vi "Read ID.vi"(8 "error in (no error)":errorcluster, 11 "8846A in":refnum<class "8846A.lvclass">) -> (0 "error out":errorcluster, 3 "8846A out":refnum<class "8846A.lvclass">)   [LabVIEW 2015, in "8846A.lvclass"]
doc: "VI used to Read Hardware ID"
uses:
  8846A.lvclass
  <instrlib>/Fluke 884X Series/Fluke 884X Series.lvlib
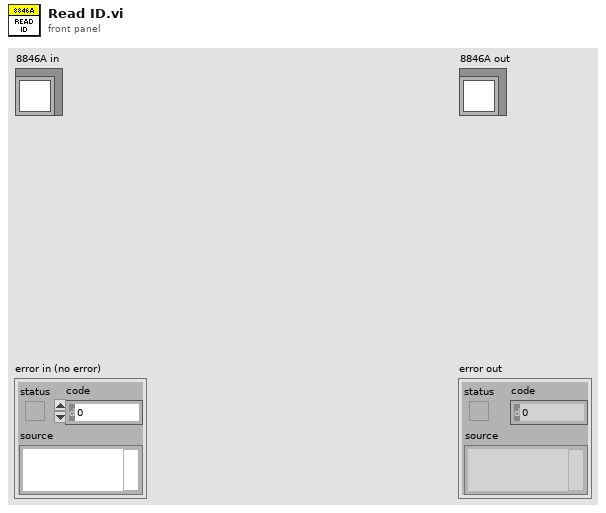
[diagram p1: front panel]
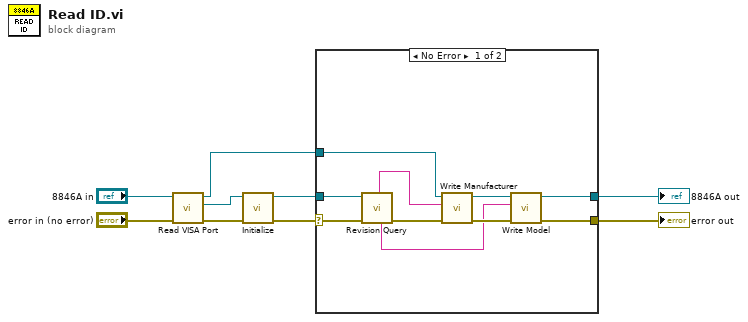
[diagram p0: block diagram]
diagram:
  n1 = call-dynamic "Read VISA Port.vi"("error in (no error)"="error in (no error)", "Device in"="8846A in") -> ("error out"=w8:errorcluster, "VISA Port"=w9:refnum<visa-resource-name>, "Device out"=w5:refnum<class "8846A.lvclass">)  [unwired: 7 in]
  n2 = call <instrlib>:"Initialize.vi"("error in (no error)"=w8, "VISA resource name"=w9) -> ("error out"=w6:errorcluster, "VISA resource name out"=w7:refnum<visa-resource-name>)  [unwired: 8 in]
  n3 = case shown="No Error" w6 {
    selector: w6 -> [w10 w20]
    tunnel: w7 -> [w19 _]
    tunnel: w5 -> [w18 w21]
    tunnel: [w12 w20] -> w1
    tunnel: [w11 w21] -> w2
    frame No Error {
      n4 = call <instrlib>:"Revision Query.vi"("error in (no error)"=w10, "VISA resource name"=w19) -> ("error out"=w16:errorcluster, "Modelo"=w13:string, "Fabricante"=w17:string)  [unwired: 4 in, 3 out]
      n5 = call-dynamic "Write Manufacturer.vi"("error in (no error)"=w16, "Manufacturer"=w17, "Device in"=w18) -> ("error out"=w15:errorcluster, "Device out"=w14:refnum<class "8846A.lvclass">)  [unwired: 7 in]
      n6 = call-dynamic "Write Model.vi"("error in (no error)"=w15, "Model"=w13, "Device in"=w14) -> ("error out"=w12:errorcluster, "Device out"=w11:refnum<class "8846A.lvclass">)  [unwired: 7 in]
    }
    frame Error {
    }
  }
  "error out" <- w1
  "8846A out" <- w2
